vi "THERMOMETER.vi"() -> (0 "temeperature":dbl)   [LabVIEW 2013]
panel:
  out "2":bool
  out "Thermomètre":dbl(slide) scale=0.0..100.0
  in  "Booléen":bool
  # "TRUE"
  # "C"
  # "F"
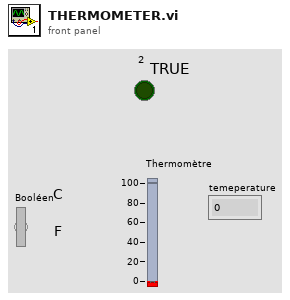
[diagram p1: front panel]
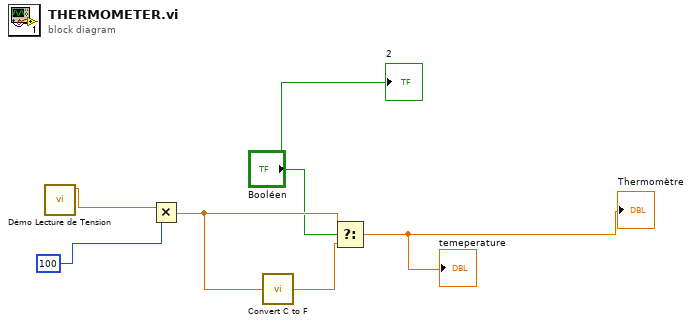
[diagram p0: block diagram]
diagram:
  n1 = call "Démo Lecture de Tension.vi"() -> ("tension"=w1:dbl)  [unwired: 6 in, 1 out]
  n2 = Multiply(x=w1, y=100) -> (x*y=w5:dbl)
  n3 = call "Convert C to F.vi"("deg. C"=w5) -> ("deg. F"=w4:dbl)
  n4 = Select(t=w5, s="Booléen", f=w4) -> (s? t:f=→"Thermomètre" →"temeperature":dbl)
  "2" <- "Booléen"
